vi "ComtManager.vi"(3 "Comment number in":i32, 4 "Comment in":string, 5 "Action":u16(ring) items=["Initialise", "Add comment", "Read Comments", "Replace comment"]) -> (0 "Comment out":string, 1 "Comments out":string[](array[string]), 2 "No of comments":i32)   [LabVIEW 2013]
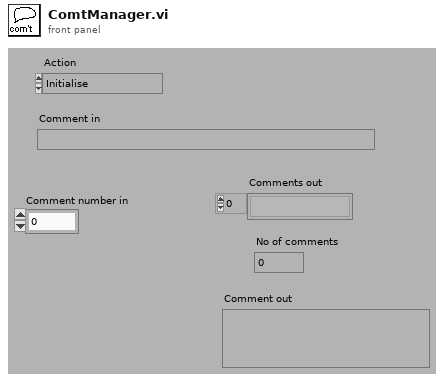
[diagram p1: front panel]
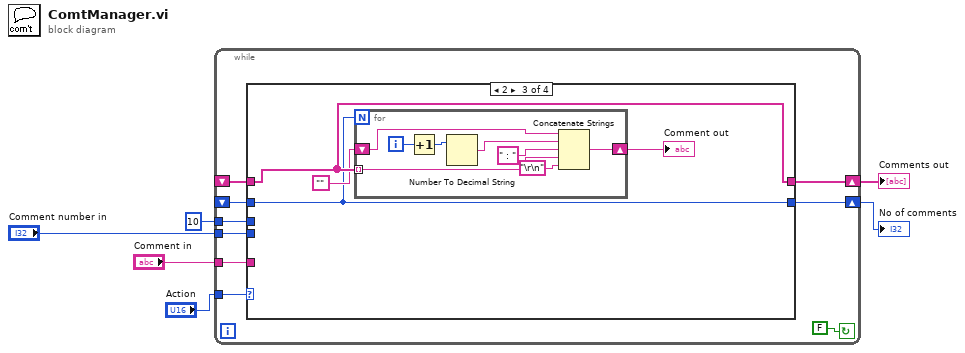
[diagram p0: block diagram]
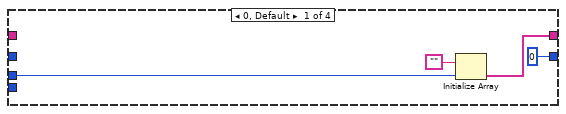
[diagram p2: hidden frame]
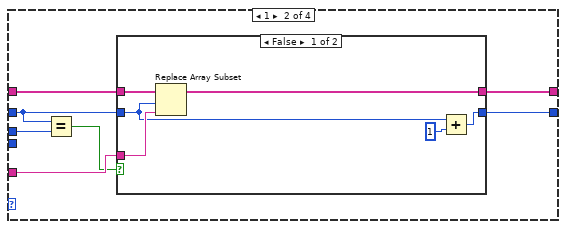
[diagram p3: hidden frame]
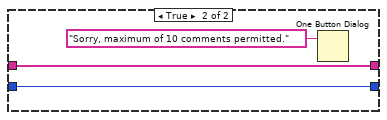
[diagram p4: hidden frame]
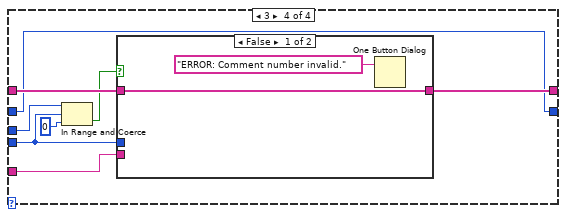
[diagram p5: hidden frame]
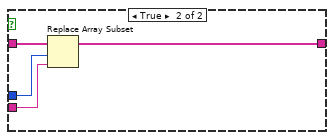
[diagram p6: hidden frame]
diagram:
  n1 = while {
    tunnel: "Comment number in" -> [w8]
    tunnel: 10 -> [w7]
    shift-left: _ -> [w10]
    shift-right: [w11] -> w3
    tunnel: "Comment in" -> [w12]
    tunnel: "Action" -> [w15]
    shift-left: _ -> [w13]
    shift-right: [w14] -> w4
    stop <- FALSE continue-if-true
    n2 = case shown="2" w15 {
      tunnel: [w18 w24 w39 w53] -> w14
      tunnel: w13 -> [_ w26 w39 w54]
      tunnel: w12 -> [_ w25 _ w55]
      tunnel: [0 w23 w36 w52] -> w11
      tunnel: w10 -> [_ w21 w36 w52]
      tunnel: w7 -> [w16 w22 _ w49]
      tunnel: w8 -> [_ _ _ w51]
      frame 0, Default {
        n3 = Initialize Array("", w16) -> (w18:string[])
      }
      frame 1 {
        n4 = Equal?(x=w21, y=w22) -> (x = y?=w20:bool)
        n5 = case shown="False" w20 {
          tunnel: w26 -> [w32 w35]
          tunnel: w25 -> [w31 _]
          tunnel: [w30 w35] -> w24
          tunnel: [w28 w34] -> w23
          tunnel: w21 -> [w27 w34]
          frame False {
            n6 = Replace Array Subset(array=w32, new element=w31, index=w27) -> (w30:string[])
            n7 = Add(x=w27, y=1) -> (x+y=w28:i32)
          }
          frame True {
            n8 = One Button Dialog(message="Sorry, maximum of 10 comments permitted.") -> ()  [unwired: 1 in, 1 out]
          }
        }
      }
      frame 2 {
        n9 = for {
          N: w36 -> [_]
          tunnel: w39 -> [w47] mode=indexing
          shift-right: [w45] -> w37
          shift-left: "" -> [w44]
          i -> [w43]
          n10 = Increment(x=w43) -> (x+1=w42:i32)
          n11 = Number To Decimal String(number=w42) -> (decimal integer string=w41:string)  [unwired: 1 in]
          n12 = Concatenate Strings(w44, w41, " : " ("Substring"), w47, "\r\n") -> (w45:string)
        }
        "Comment out" <- w37
      }
      frame 3 {
        n13 = In Range and Coerce(upper limit=w49, x=w51, lower limit=0) -> (In Range?=w48:bool)  [unwired: 1 out]
        n14 = case shown="False" w48 {
          tunnel: w55 -> [_ w61]
          tunnel: w54 -> [w57 w60]
          tunnel: [w57 w59] -> w53
          tunnel: w51 -> [_ w58]
          frame False {
            n15 = One Button Dialog(message="ERROR: Comment number invalid.") -> ()  [unwired: 1 in, 1 out]
          }
          frame True {
            n16 = Replace Array Subset(array=w60, new element=w61, index=w58) -> (w59:string[])
          }
        }
      }
    }
  }
  "Comments out" <- w4
  "No of comments" <- w3
